vi "Start Lock-In Path.vi"(7 "instance":i32, 8 "error in":errorcluster, 10 "config":T1, 11 "fpga session in":refnum<k20>) -> (0 "error out":errorcluster, 3 "fpga session out":refnum<k20>)   [LabVIEW 2017, in "Lock-In Amplifier Example Host.lvlib"]
uses:
  Lock-In Amplifier Example Host.lvlib
  lock-in settings.ctl
  fpga type.ctl
  <vilib>/Utility/error.llb/Error Cluster From Error Code.vi
  <vilib>/rvi/errors/niLvFpgaAdjustHostInterfaceError.vi
  <instrlib>/_niInstr/Streaming/v1/Host/Public/Start Continuous Stream.vi
  <vilib>/rvi/interface/nirviReadWriteControl/nirviReadWriteControl.xnode
  NiFpgaLv.dll
  <vilib>/rvi/interface/Simulation/niFpgaSimulationCallBeginRW.vi
  <instrlib>/_niInstr/Streaming/v1/Host/niInstr Streaming v1 Host.lvlib
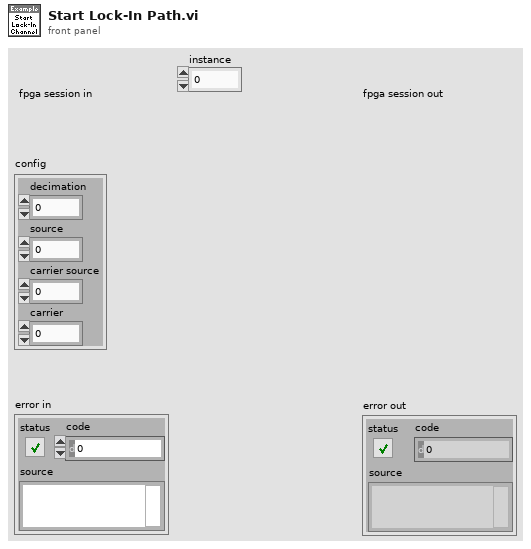
[diagram p1: front panel]
types:
  T1 = typedef "Lock-In Amplifier Example Host.lvlib/lock-in settings.ctl" = cluster{"decimation":i32, "source":i32, "carrier source":i32, "carrier":dbl}
  T2 = typedef "Lock-In Amplifier Example Host.lvlib/fpga type.ctl" = refnum<k20>
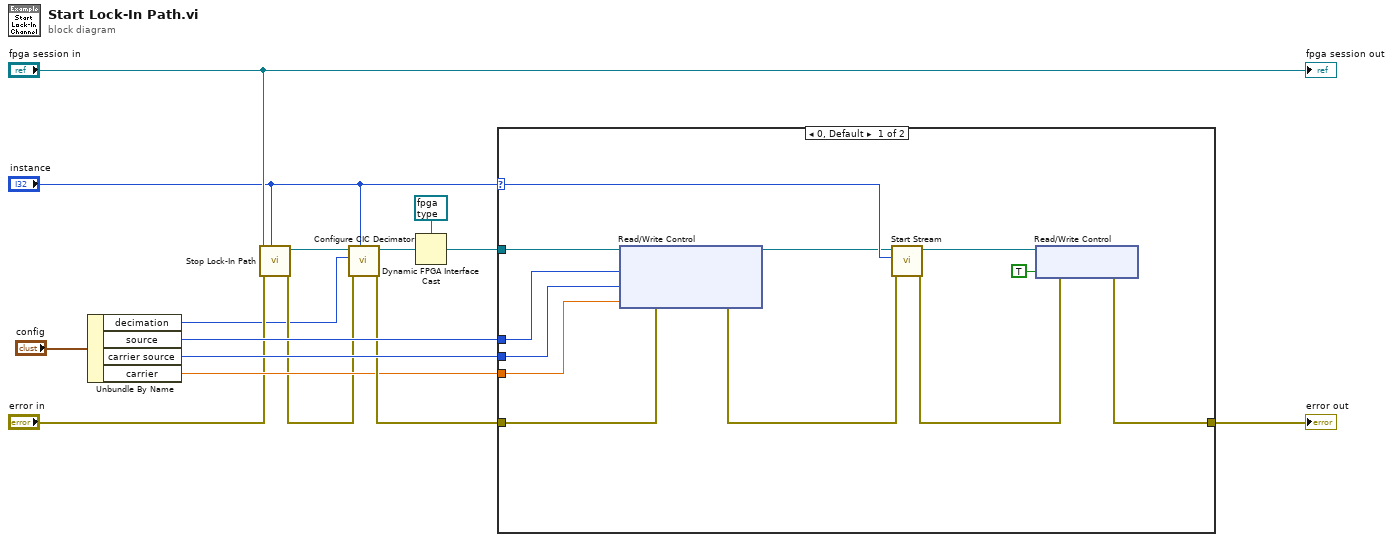
[diagram p0: block diagram]
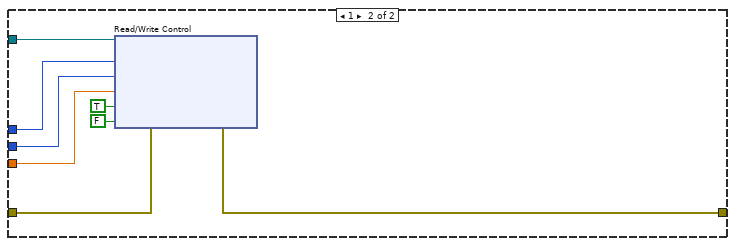
[diagram p2: hidden frame]
diagram:
  n1 = Unbundle By Name("config") -> ("decimation"=w1:i32, "source"=w11:i32, "carrier source"=w10:i32, "carrier"=w7:dbl)
  n2 = call "Stop Lock-In Path.vi"("instance"="instance", "error in"="error in", "fpga session in"="fpga session in") -> ("error out"=w4:errorcluster, "fpga session out"=w6:refnum<k20>)  [unwired: 7 in]
  n3 = call "Configure CIC Decimator.vi"("index"="instance", "error in"=w4, "decimation"=w1, "fpga session in"=w6) -> ("error out"=w8:errorcluster, "fpga session out"=w13:refnum<k20>)  [unwired: 6 in]
  n4 = Dynamic FPGA Interface Cast(Session In=T2 refnum ("fpga type"), Type=w13) -> (Session Out=w12:T2)
  n5 = case shown="0, Default" "instance" {
    selector: "instance" -> [w21 _]
    tunnel: w12 -> [w27 w35]
    tunnel: w11 -> [w26 w34]
    tunnel: w10 -> [w25 w33]
    tunnel: [w20 w28] -> w9
    tunnel: w8 -> [w23 w29]
    tunnel: w7 -> [w24 w32]
    frame 0, Default {
      n6 = xnode "Read/Write Control"("FPGA VI Reference In"=w27, "error in"=w23, "lock-in.channel select 0"=w26, "lock-in.carrier select 0"=w25, "lock-in.carrier 0"=w24) -> ("FPGA VI Reference Out"=w19:T2, "error out"=w18:errorcluster)
      n7 = call-poly <instrlib>:"Start Stream.vi"("error in (no error)"=w18, "stream index"=w21, "refnum in"=w19) -> ("error out"=w17:errorcluster, "refnum out"=w16:T2)  [unwired: 7 in]
      n8 = xnode "Read/Write Control"("FPGA VI Reference In"=w16, "error in"=w17, "lock-in.enable 0"=TRUE) -> ("error out"=w20:errorcluster)  [unwired: 1 out]
    }
    frame 1 {
      n9 = xnode "Read/Write Control"("FPGA VI Reference In"=w35, "error in"=w29, "lock-in.channel select 1"=w34, "lock-in.carrier select 1"=w33, "lock-in.carrier 1"=w32, "lock-in.reset 1"=TRUE ("lock-in.reset 0"), "lock-in.reset 1"=FALSE ("lock-in.reset 0")) -> ("error out"=w28:errorcluster)  [unwired: 1 out]
    }
  }
  "error out" <- w9
  "fpga session out" <- "fpga session in"
